vi "Ex3.vi"() -> ()   [LabVIEW 2010]
uses:
  ROS/Code/SubVIs/BaxterButtons.ctl
  ROS/Code/SubVIs/DigitalIOComponents.ctl
panel:
  in  "stop":bool
  out "Changed_IO":T2(array[cluster])
  out "Left ITB":T3
  # "Hitting the long buttons on his wrist toggles the lights on his arms"
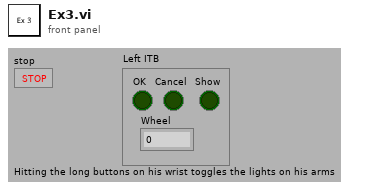
[diagram p1: front panel]
types:
  T1 = typedef "DigitalIOComponents.ctl" = enum16{"left_lower_cuff", "right_lower_cuff", "left_lower_button", "right_lower_button", "left_upper_button", "right_upper_button", "left_shoulder_button", "right_shoulder_button"}
  T2 = cluster{"Component":T1, "state":i8, "is input only":bool}[]
  T3 = cluster{"OK":bool, "Cancel":bool, "Show":bool, "Wheel":u8}
  T4 = typedef "BaxterButtons.ctl" = enum16{"left_itb", "right_itb", "torso_left_itb", "torso_right_itb"}
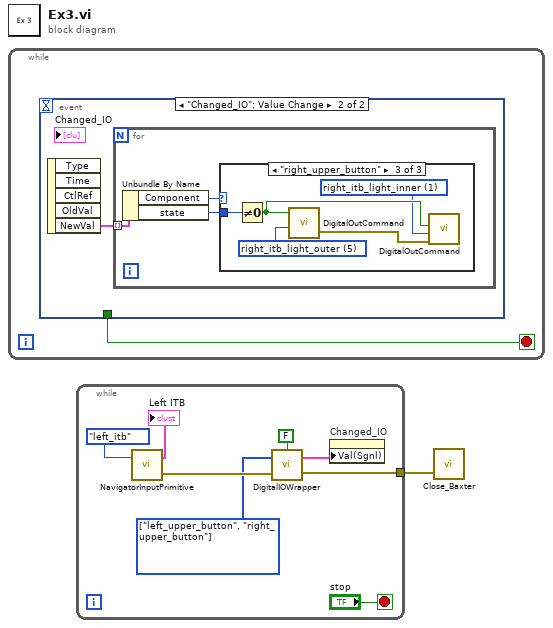
[diagram p0: block diagram]
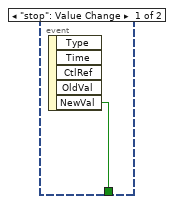
[diagram p2: hidden frame]
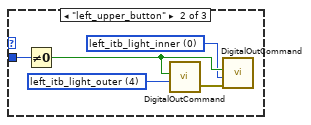
[diagram p4: hidden frame]
diagram:
  n1 = while {
    stop <- w2 stop-if-true
    n2 = event shown="[1] \"Changed_IO\": Value Change" {
      selector: _ -> [_ _]
      dyn-events: _ -> [_ _]
      timeout: _ -> [_ _]
      tunnel: [w3 _] -> w2
      event "stop": Value Change {
        n3 = event-data() -> ("NewVal"=w3:bool)  [unwired: 1 in, 4 out]
      }
      event "Changed_IO": Value Change {
        n4 = event-data() -> ("NewVal"=w4:T2)  [unwired: 1 in, 4 out]
        n5 = for {
          tunnel: w4 -> [w7] mode=indexing
          n6 = Unbundle By Name(w7) -> ("Component"=w6:T1, "state"=w5:i8)
          n7 = case shown="\"right_upper_button\"" w6 {
            tunnel: w5 -> [_ w12 w17]
            frame Default {
            }
            frame "left_upper_button" {
              w8 = u16 0 items=["left_itb_light_inner", "right_itb_light_inner", "torso_left_itb_light_inner", "torso_right_itb_light_inner", "left_itb_light_outer", "right_itb_light_outer", "torso_left_itb_light_outer", "torso_right_itb_light_outer", ""] ("Component ID")
              w11 = u16 4 items=["left_itb_light_inner", "right_itb_light_inner", "torso_left_itb_light_inner", "torso_right_itb_light_inner", "left_itb_light_outer", "right_itb_light_outer", "torso_left_itb_light_outer", "torso_right_itb_light_outer", ""] ("Component ID")
              n8 = Not Equal To 0?(x=w12) -> (x != 0?=w9:bool)
              n9 = call "DigitalOutCommand.vi"("Component ID"=w11, "State"=w9) -> ("error out"=w10:errorcluster)  [unwired: 3 in]
              n10 = call "DigitalOutCommand.vi"("error in"=w10, "Component ID"=w8, "State"=w9) -> ()  [unwired: 2 in, 1 out]
            }
            frame "right_upper_button" {
              w14 = u16 1 items=["left_itb_light_inner", "right_itb_light_inner", "torso_left_itb_light_inner", "torso_right_itb_light_inner", "left_itb_light_outer", "right_itb_light_outer", "torso_left_itb_light_outer", "torso_right_itb_light_outer", ""] ("Component ID")
              w16 = u16 5 items=["left_itb_light_inner", "right_itb_light_inner", "torso_left_itb_light_inner", "torso_right_itb_light_inner", "left_itb_light_outer", "right_itb_light_outer", "torso_left_itb_light_outer", "torso_right_itb_light_outer", ""] ("Component ID")
              n11 = Not Equal To 0?(x=w17) -> (x != 0?=w15:bool)
              n12 = call "DigitalOutCommand.vi"("Component ID"=w16, "State"=w15) -> ("error out"=w13:errorcluster)  [unwired: 3 in]
              n13 = call "DigitalOutCommand.vi"("error in"=w13, "Component ID"=w14, "State"=w15) -> ()  [unwired: 2 in, 1 out]
            }
          }
        }
      }
    }
  }
  n14 = while {
    tunnel: [w20] -> w1
    stop <- "stop" stop-if-true
    w19 = T1[] [enum."left_upper_button", enum."right_upper_button"] items=["left_lower_cuff", "right_lower_cuff", "left_lower_button", "right_lower_button", "left_upper_button", "right_upper_button", "left_shoulder_button", "right_shoulder_button"] ("Component IDs")
    n15 = call "NavigatorInputPrimitive.vi"("Component"=BaxterButtons."left_itb") -> ("error out"=w21:errorcluster, "Navigator Inputs"=→"Left ITB":T3)  [unwired: 2 in]
    n16 = call "DigitalIOWrapper.vi"("error in"=w21, "Component IDs"=w19, "True Only (T)"=FALSE) -> ("error out"=w20:errorcluster, "Changed_IO"=w18:T2)
    n17 = property on="Changed_IO" class="Arr (strict)"("Val(Sgnl)"=w18) -> ()  [unwired: 2 in, 2 out]
  }
  n18 = call "Close_Baxter.vi"("error in"=w1) -> ()  [unwired: 3 in, 1 out]
